vi "readPress06.vi"() -> (0 "P":dbl)   [LabVIEW 2011]
doc: "The Basic Serial Read and Write example performs a Serial Port Read, a Serial Port Write, or a combination of these actions. The user selects the actions (read or write) on the front panel. If both are selected, the VI will write the data first, read data, and then close the VISA session that is opened to the port. This VI will wait until the specified number of bytes is received at the port or until a termination character is read.\n\nINSTRUCTIONS:\n1) Select the serial resource and configuration parameters (baud rate, data bits, parity, stop bits, flow control).\n2) Select the operations to be performed. \n3) Connect the serial port to your device. If no device is available, perform a loopback test by doing one of the following. Short pins 2 and 3 on a RS-232 cable or short pin 4 to pin 8 and pin 5 to pin 9 on a RS-485/422 cable. \n4) Run the VI to see the data read. (The \"read string\" will match the \"string to write\" if a loopback test was performed.)\n\nNote: The parameters set for the serial port must match the parameters of the connected instrument or device. In this example, the bytes to read parameter specifies the number of bytes that the serial port reads. If there were more bytes at the port than the number specified in bytes to read, those bytes would not be read. Also, if you specify to read more bytes than the number of bytes actually read, you might receive a timeout error message.\n\nOn the block diagram, the Configure Serial Port VI sets the configuration parameters. The front panel displays the controls used to configure the basic parameters, such as baud rate, data bits, and parity. Constants configure the other parameters the user probably does not need set. After the VISA Configure Serial Port VI opens the VISA session and configures the port, the VI passes the VISA resource name to other VIs that perform operations on that VISA resource. The VISA Write function sends a command to the serial device and the VISA Read function returns data based on the command. The VISA Close function then closes the reference to the serial device. It is important to close the reference; otherwise communication through with that port through protocols other than VISA might not be possible."
uses:
  <vilib>/Instr/_visa.llb/VISA Configure Serial Port (Instr).vi
panel:
  in  "Tab Control":enum32{"I/O", "AdapTorr"}(tab)
  in  "VISA resource name":refnum<visa-resource-name>="COM1"
  in  "baud rate":u32=9600
  in  "data bits":u16=8 min=5 max=8 step=1
  in  "parity":u16(ring) items=["None", "Odd", "Even", "Mark", "Space"]
  in  "stop bits":u16(ring)=20 items=["2"=10, "1.5"=15, "2.0"=20]
  in  "flow control":u16(ring) items=["None"=0, "XON/XOFF"=1, "RTS/CTS"=2, "DTR/DSR"=4]
  in  "delay before read (ms)":u32=500
  in  "head range (Torr)":i32=1000
  out "P(Torr)":string
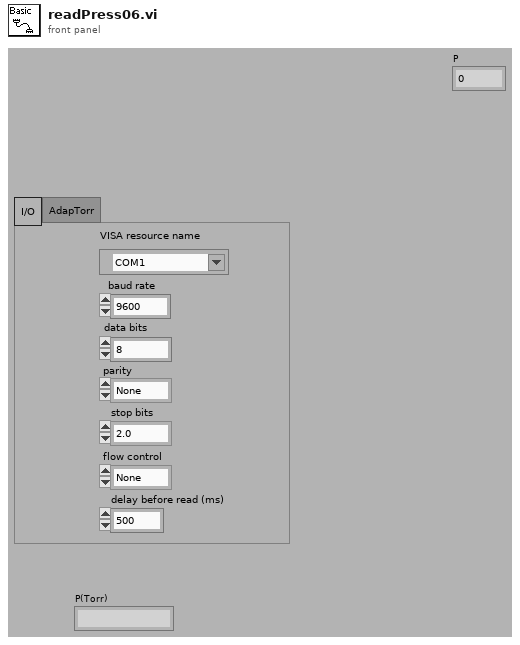
[diagram p1: front panel]
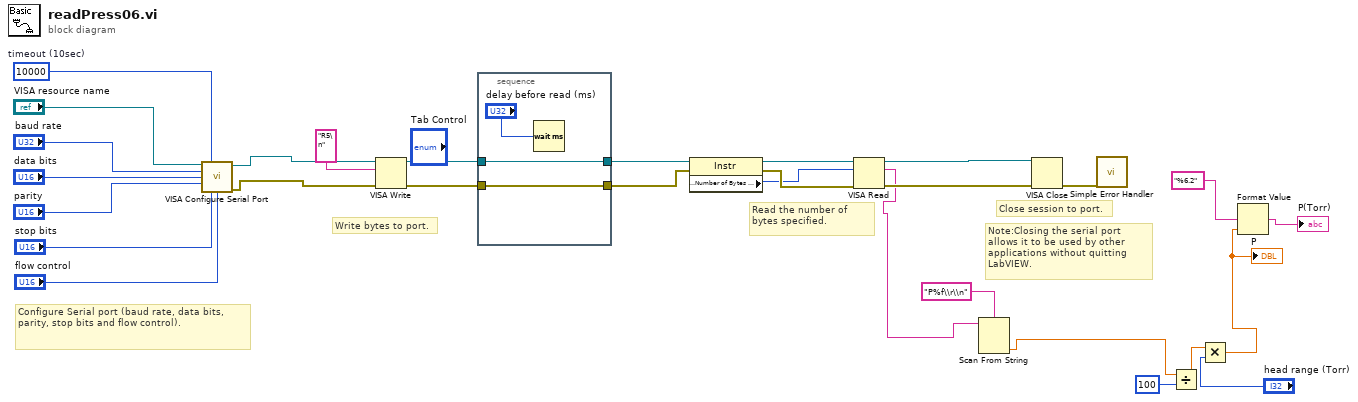
[diagram p0: block diagram]
diagram:
  w23 = u32 10000  # timeout (10sec)
  # "Write bytes to port."
  # "Read the number of bytes specified."
  # "Note:Closing the serial port allows it to be used by other applications without quitting LabVIEW."
  # "Configure Serial port (baud rate, data bits, parity, stop bits and flow control)."
  # "Close session to port."
  n1 = call-poly "VISA Configure Serial Port"("VISA resource name"="VISA resource name", "timeout (10sec)"=w23, "baud rate (9600)"="baud rate", "data bits (8)"="data bits", "parity (0:none)"="parity", "stop bits (10: 1 bit)"="stop bits", "flow control (0:none)"="flow control") -> ("VISA resource name out"=w15:refnum<visa-resource-name>, "error out"=w14:errorcluster)  [unwired: 2 in, 5 out]
  n2 = VISA Write(VISA resource name=w15, write buffer="R5\n" ("string to write"), error in (no error)=w14) -> (VISA resource name out=w17:refnum<visa-resource-name>, error out=w19:errorcluster)  [unwired: 1 out]
  n3 = stacked-sequence {
    tunnel: w19 -> [w32]
    tunnel: [w32] -> w18
    tunnel: w17 -> [w31]
    tunnel: [w31] -> w16
    frame #0 {
      n4 = Wait (ms)(milliseconds to wait="delay before read (ms)") -> ()  [unwired: 1 out]
    }
  }
  n5 = property class="Instr"(reference=w16, error in=w18) -> (reference out=w10:refnum<visa-resource-name>, error out=w9:errorcluster, "Serial Settings:Number of Bytes at Serial Port"=w8:u32)
  n6 = VISA Read(VISA resource name=w10, byte count=w8, error in (no error)=w9) -> (VISA resource name out=w26:refnum<visa-resource-name>, read buffer=w6:string, error out=w27:errorcluster)  [unwired: 1 out]
  n7 = Scan From String(format string="P%f\\r\\n", input string=w6) -> (output 1=w5:dbl)  [unwired: 3 in, 3 out]
  n8 = VISA Close(VISA resource name=w26, error in (no error)=w27) -> (error out=w25:errorcluster)
  n9 = call <vilib>:"Simple Error Handler.vi"("error in (no error)"=w25) -> ()  [unwired: 1 in, 8 out]
  n10 = Divide(x=w5, y=100) -> (x/y=w11:dbl)
  n11 = Multiply(x=w11, y="head range (Torr)") -> (x*y=w3:dbl)
  "P" <- w3
  n12 = Format Value(format string="%6.2", value (0)=w3) -> (output string=→"P(Torr)":string)  [unwired: 1 in]
